vi "Get Sensor Mode.vi"(8 "error in (no error)":errorcluster) -> (0 "error out":errorcluster, 3 "Sensor Mode?":bool)   [LabVIEW 2013]
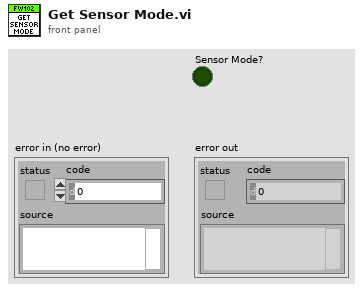
[diagram p1: front panel]
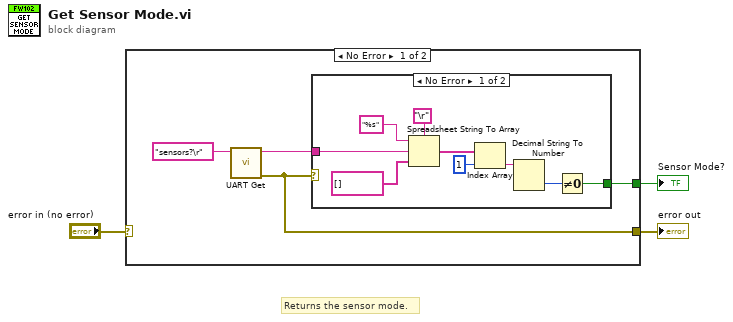
[diagram p0: block diagram]
diagram:
  # "Returns the sensor mode."
  n1 = case shown="No Error" "error in (no error)" {
    selector: "error in (no error)" -> [_ w17]
    tunnel: [w7 _] -> w3
    tunnel: [w4 w17] -> w2
    frame No Error {
      n2 = call "UART Get.vi"("Command"="sensors?\r" ("Input Command String")) -> ("error out"=w4:errorcluster, "Returned String"=w5:string)  [unwired: 9 in]
      n3 = case shown="No Error" w4 {
        tunnel: w5 -> [w16 _]
        tunnel: [w8 _] -> w7
        frame No Error {
          n4 = Spreadsheet String To Array(delimiter (Tab)="\r", format string="%s", spreadsheet string=w16, array type (2D Dbl)=string[] []) -> (array=w12:string[])
          n5 = Index Array(array=w12, index=1) -> (element=w10:string)
          n6 = Decimal String To Number(string=w10) -> (number=w9:i32)  [unwired: 2 in, 1 out]
          n7 = Not Equal To 0?(x=w9) -> (x != 0?=w8:bool)
        }
        frame Error {
        }
      }
    }
    frame Error {
    }
  }
  "error out" <- w2
  "Sensor Mode?" <- w3
